vi "SLM Control.vi"() -> ()   [LabVIEW 2014]
uses:
  Controls/SLM General Settings.ctl
  Controls/Holo Settings.ctl
panel:
  in  "Exit":bool
  in  "Holo 2":T1={"Top Hat"=FALSE, "Modes"=[], "Vortex"=FALSE, "Clockwise"=FALSE, "X"=-200.0, "Y"=0.0, "Holo ON"=TRUE, "Scan"=FALSE} {"Modes"."Amplititute" step=0.05}
  out "Intensity Graph":u8[][](graph)
  in  "Holo 1":T1={"Top Hat"=FALSE, "Modes"=[], "Vortex"=FALSE, "Clockwise"=FALSE, "X"=200.0, "Y"=0.0, "Holo ON"=TRUE, "Scan"=FALSE} {"Modes"."Amplititute" step=0.05}
  in  "General settings":T2={"Holo size (pixels)"=300, "Top hat radius"=0.5, "Number of modes"=20, "Bkg gradient X"=40.0, "Bkg gradient Y"=40.0, "Flat"=FALSE, "Mode Matrix"=1} {"Mode Matrix" items=["Unit Matrix", "Unit Matrix_AbbNames"]; "Top hat radius" min=0.0 max=0.99 step=0.05 format="%.3f"}
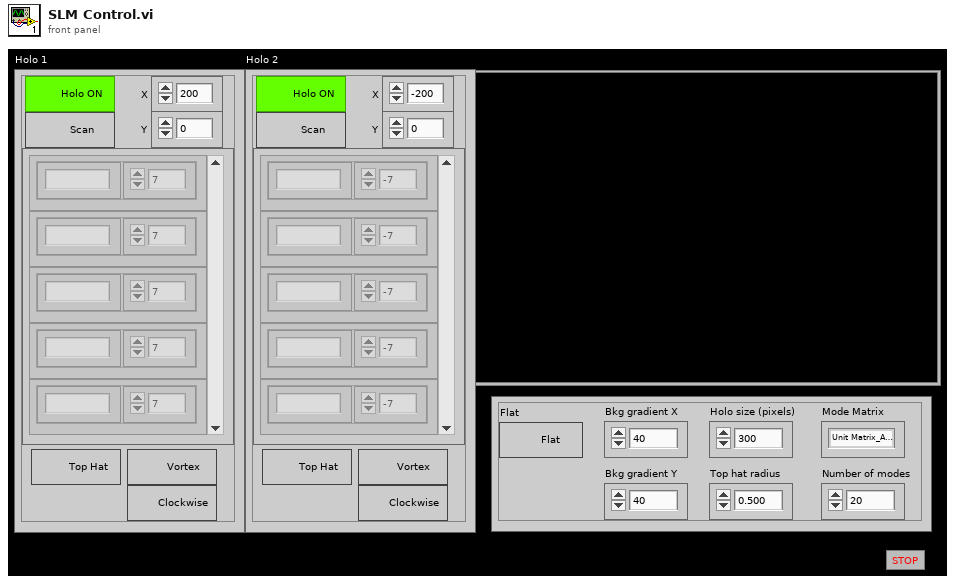
[diagram p1: front panel]
types:
  T1 = typedef "Holo Settings.ctl" = cluster{"Top Hat":bool, "Modes":cluster{"Mode ID":string, "Amplititute":dbl}[], "Vortex":bool, "Clockwise":bool, "X":dbl, "Y":dbl, "Holo ON":bool, "Scan":bool}
  T2 = typedef "SLM General Settings.ctl" = cluster{"Holo size (pixels)":i32, "Top hat radius":dbl, "Number of modes":i32, "Bkg gradient X":dbl, "Bkg gradient Y":dbl, "Flat":bool, "Mode Matrix":u16}
  T3 = cluster{"Holo size (pixels)":bool, "Top hat radius":bool, "Number of modes":bool, "Bkg gradient X":bool, "Bkg gradient Y":bool, "Flat":bool, "Mode Matrix":bool}
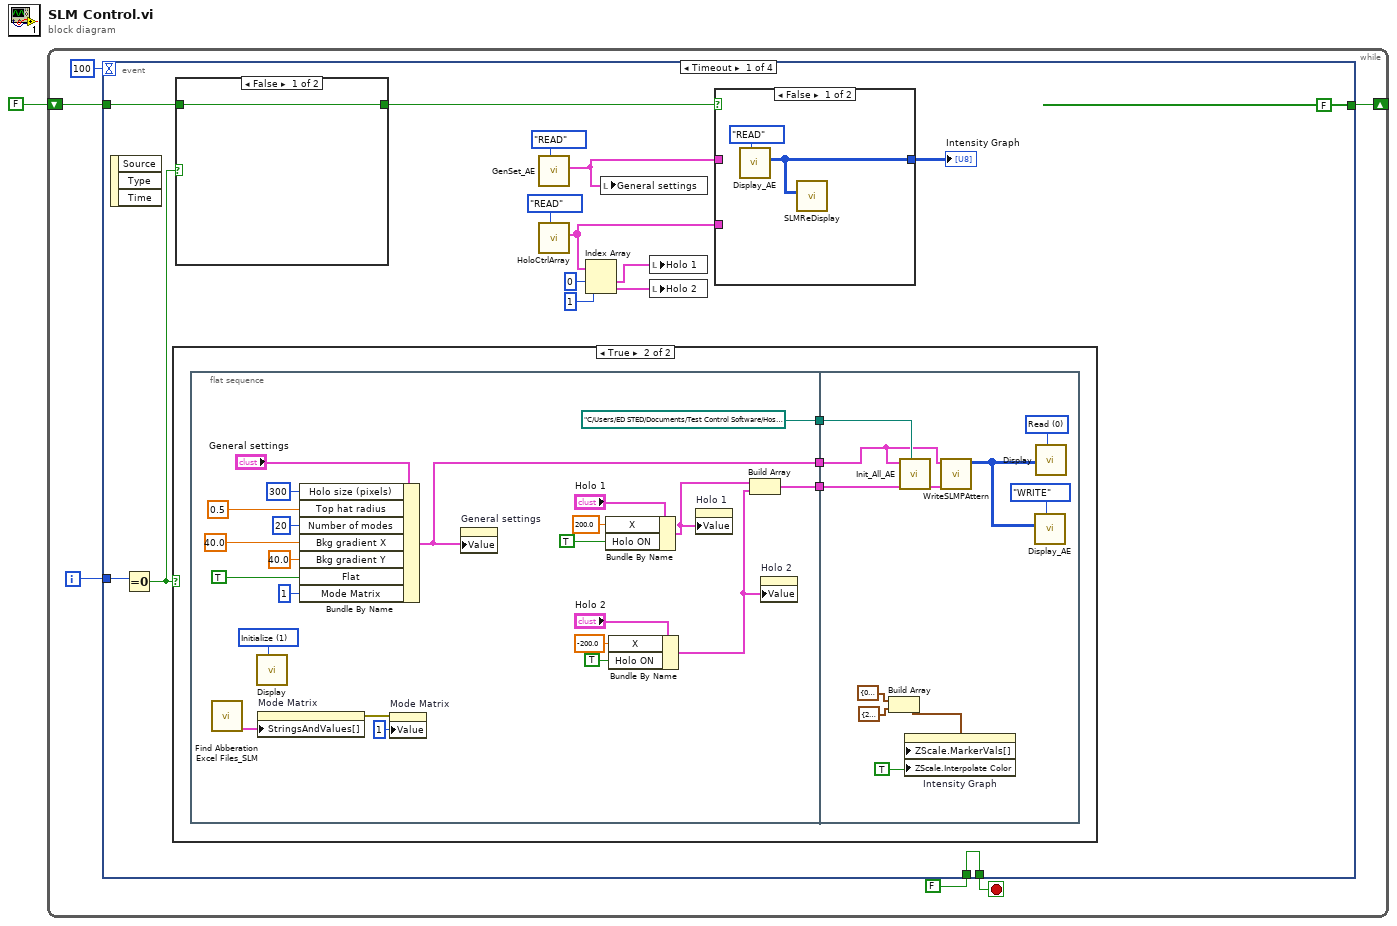
[diagram p0: block diagram]
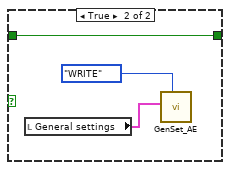
[diagram p2: hidden frame]
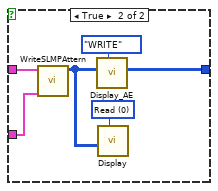
[diagram p3: hidden frame]
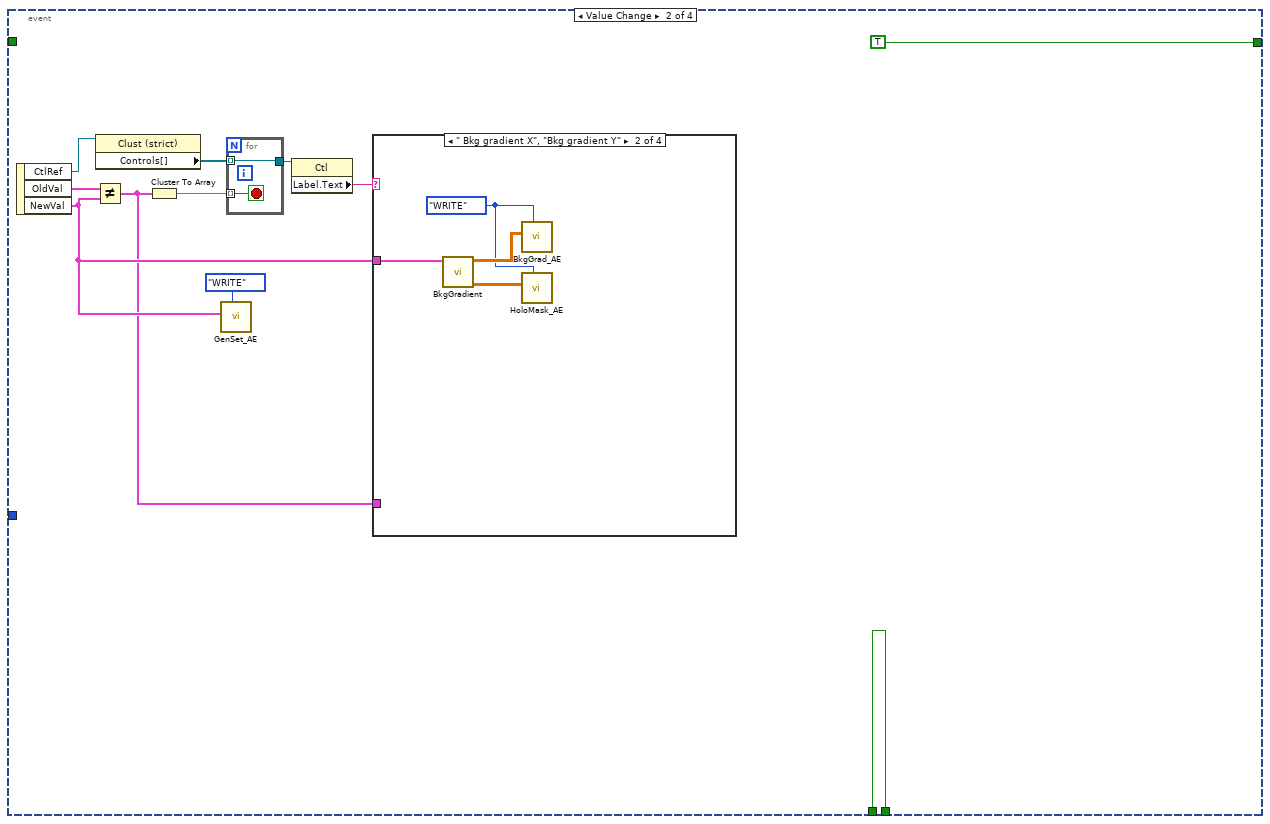
[diagram p5: hidden frame]
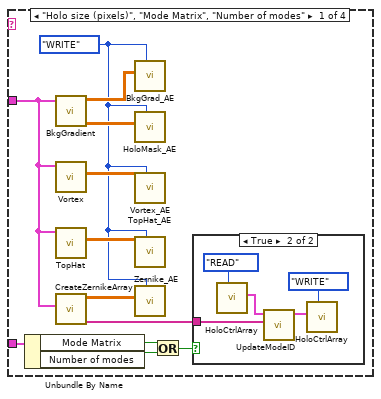
[diagram p6: hidden frame]
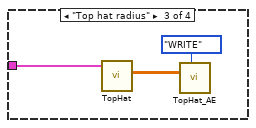
[diagram p8: hidden frame]
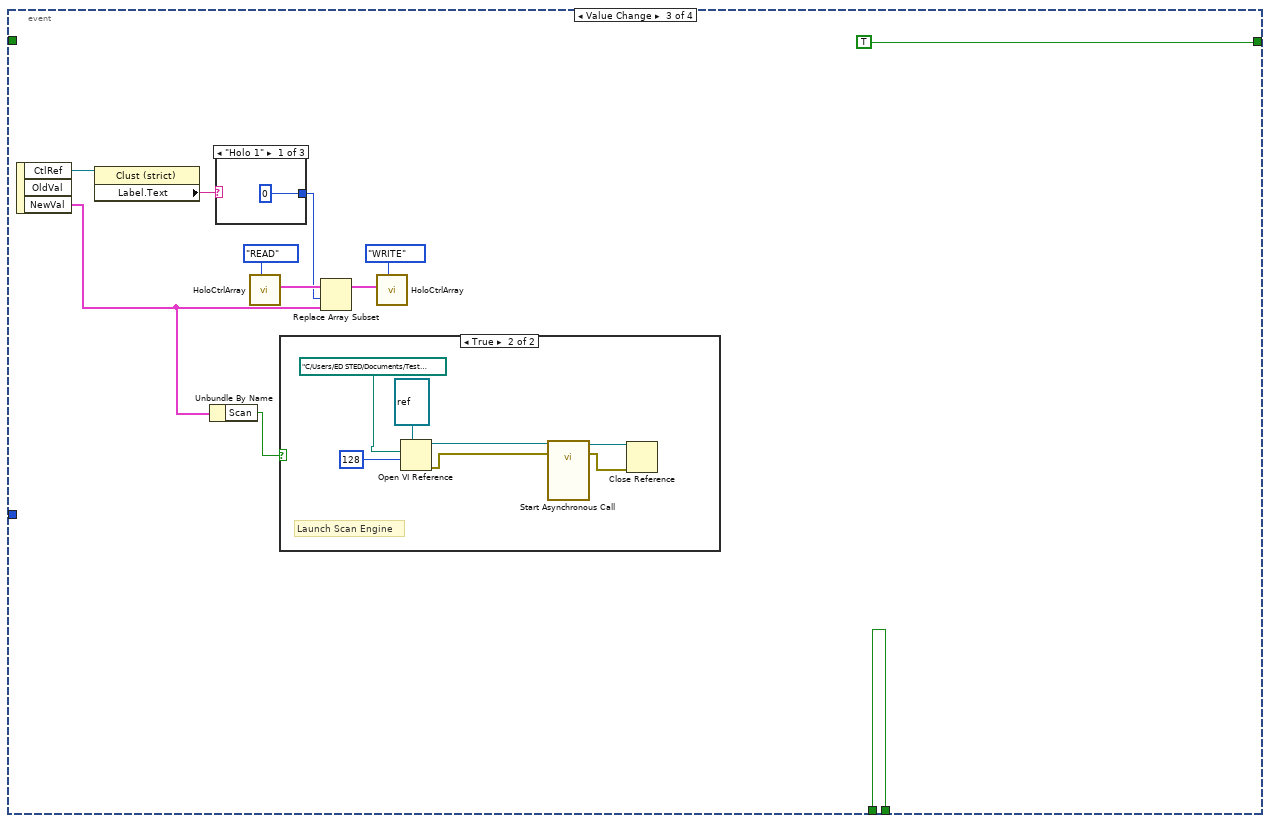
[diagram p10: hidden frame]
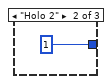
[diagram p12: hidden frame]
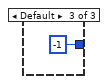
[diagram p13: hidden frame]
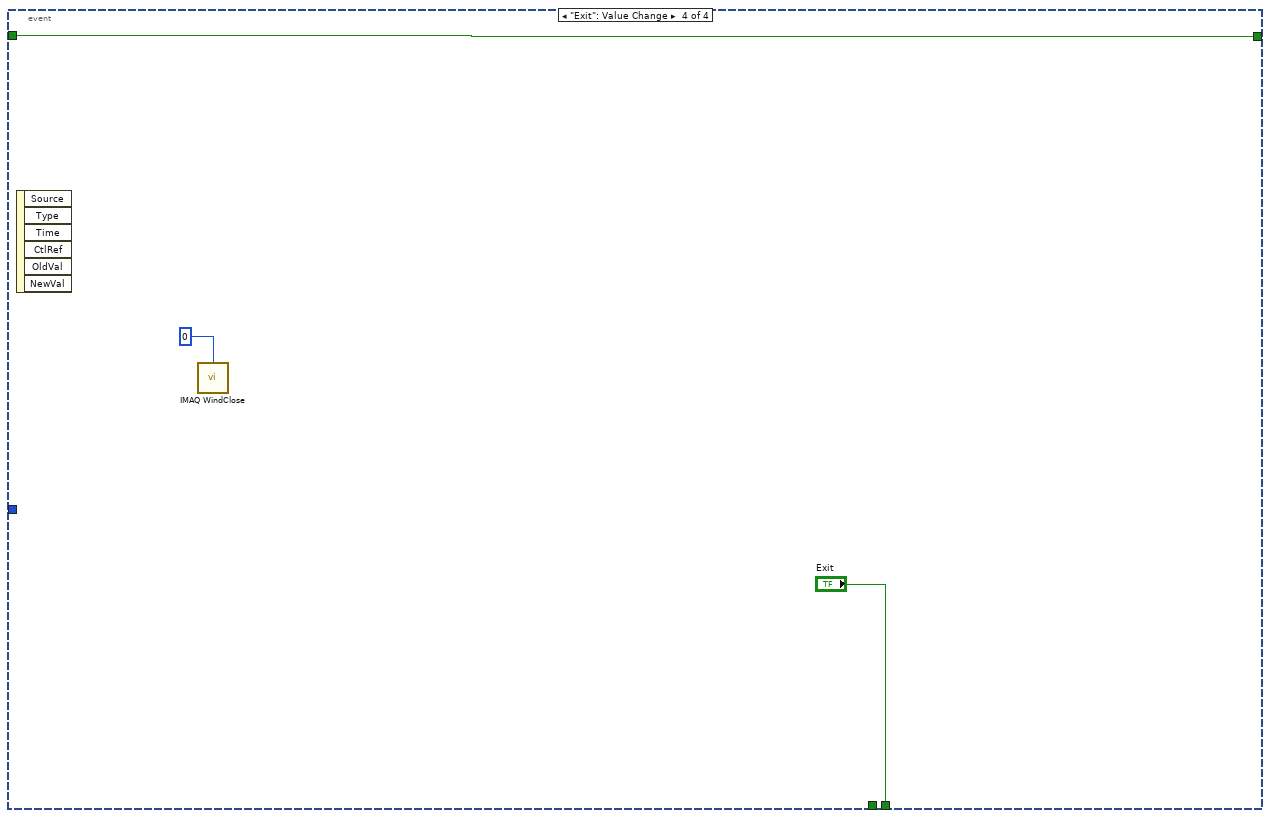
[diagram p14: hidden frame]
diagram:
  n1 = while {
    shift-right: [w4] -> _
    shift-left: FALSE -> [w5]
    i -> [w6]
    stop <- w3 stop-if-true
    n2 = event shown="[0] Timeout" {
      selector: _ -> [_ _ _ _]
      dyn-events: _ -> [_ _ _ _]
      timeout: 100 -> [_ _ _ _]
      tunnel: w6 -> [w22 _ _ _]
      tunnel: w5 -> [w10 _ _ w131]
      tunnel: [FALSE TRUE TRUE w131] -> w4
      tunnel: [w11 w73 w111 "Exit"] -> w3
      tunnel: FALSE -> [w11 w73 w111 _]
      event Timeout {
        n3 = event-data() -> ()  [unwired: 1 in, 3 out]
        n4 = Equal To 0?(x=w22) -> (x = 0?=w8:bool)
        n5 = case shown="True" w8 {
          frame False {
          }
          frame True {
            n6 = flat-sequence {
              tunnel: [w40] -> w37
              tunnel: [w56] -> w36
              tunnel: [path "C:/Users/ED STED/Documents/Test Control Software/Host VIs/SLM/Flatness Correction LSH0700935/CAL_LSH0700935_770nm.bmp" ("Flat File Path")] -> w35
              tunnel: w37 -> [w63]
              tunnel: w36 -> [w71]
              tunnel: w35 -> [w68]
              frame #0 {
                w57 = u16 1 items=["Read", "Initialize"] ("Action")
                n7 = call "Find Abberation Excel Files_SLM.vi"() -> ("Ring Menu"=w60:cluster{"result string":string, i32}[])  [unwired: 10 in, 1 out]
                n8 = call "Display.vi"("Action"=w57) -> ()  [unwired: 10 in, 1 out]
                n9 = property on="Mode Matrix" class="Ring (strict)"("StringsAndValues[]"=w60) -> (error out=w59:errorcluster)  [unwired: 2 in, 1 out]
                n10 = Bundle By Name(cluster="General settings", "Holo size (pixels)"=300, "Top hat radius"=0.5, "Number of modes"=20, "Bkg gradient X"=40.0, "Bkg gradient Y"=40.0, "Flat"=TRUE, "Mode Matrix"=u16 1) -> (w40:T2)
                n11 = property on="Mode Matrix" class="Ring (strict)"(error in=w59, "Value"=u16 1) -> ()  [unwired: 1 in, 2 out]
                n12 = property on="General settings" class="Clust (strict)"("Value"=w40) -> ()  [unwired: 2 in, 2 out]
                n13 = Bundle By Name(cluster="Holo 1", "X"=200.0, "Holo ON"=TRUE) -> (w44:T1)
                n14 = Bundle By Name(cluster="Holo 2", "X"=-200.0, "Holo ON"=TRUE) -> (w41:T1)
                n15 = property on="Holo 1" class="Clust (strict)"("Value"=w44) -> ()  [unwired: 2 in, 2 out]
                n16 = Build Array(w44, w41) -> (w56:T1[])
                n17 = property on="Holo 2" class="Clust (strict)"("Value"=w41) -> ()  [unwired: 2 in, 2 out]
              }
              frame #1 {
                w70 = u16 0 items=["Read", "Initialize"] ("Action")
                n18 = Build Array(cluster{dbl, u32} {0.0, 0}, cluster{dbl, u32} {255.0, 16448250}) -> (w64:cluster{dbl, u32}[])
                n19 = call "Init_All_AE.vi"("Flat File Path"=w68, "HoloArray In"=w71, "General settings"=w63) -> ("Holo Array Out"=w69:T1[])  [unwired: 8 in]
                n20 = property on="Intensity Graph" class="IntGraph (strict)"("ZScale.MarkerVals[]"=w64, "ZScale.Interpolate Color"=TRUE ("Z Scale.Interpolate Color")) -> ()  [unwired: 2 in, 2 out]
                n21 = call "WriteSLMPAttern.vi"("Holo Array"=w69, "General settings"=w63) -> ("Display Array"=w61:u8[][])  [unwired: 9 in]
                n22 = call "Display_AE.vi"("Action"=enum16{"READ", "WRITE"}."WRITE", "Display Array In"=w61) -> ()  [unwired: 9 in, 1 out]
                n23 = call "Display.vi"("Action"=w70, "displayed matrix"=w61) -> ()  [unwired: 9 in, 1 out]
              }
            }
          }
        }
        n24 = case shown="False" w8 {
          tunnel: w10 -> [w23 w26]
          tunnel: [w23 w26] -> w9
          frame False {
          }
          frame True {
            n25 = local read "General settings"() -> (w24:T2)
            n26 = call "GenSet_AE.vi"("Enum"=enum16{"READ", "WRITE"}."WRITE", "General settings"=w24) -> ()  [unwired: 9 in, 1 out]
          }
        }
        n27 = call "GenSet_AE.vi"("Enum"=enum16{"READ", "WRITE"}."READ") -> ("General settings Out"=w18:T2)  [unwired: 10 in]
        n28 = call "HoloCtrlArray.vi"("Action"=enum16{"READ", "WRITE"}."READ") -> ("Holo Array Out"=w17:T1[])  [unwired: 10 in]
        n29 = Index Array(array=w17, index #1=0 ("index"), index #2=1 ("index")) -> (element #1=w16:T1, element #2=w15:T1)
        n30 = local write "General settings"(w18) -> ()
        n31 = local write "Holo 1"(w16) -> ()
        n32 = local write "Holo 2"(w15) -> ()
        n33 = case shown="False" w9 {
          tunnel: w18 -> [_ w34]
          tunnel: w17 -> [_ w33]
          tunnel: [w27 w29] -> w12
          frame False {
            n34 = call "Display_AE.vi"("Action"=enum16{"READ", "WRITE"}."READ") -> ("Display Array Out"=w27:u8[][])  [unwired: 10 in]
            n35 = call "SLMReDisplay.vi"("displayed matrix"=w27) -> ()  [unwired: 11 in]
          }
          frame True {
            w32 = u16 0 items=["Read", "Initialize"] ("Action")
            n36 = call "WriteSLMPAttern.vi"("Holo Array"=w33, "General settings"=w34) -> ("Display Array"=w31:u8[][])  [unwired: 9 in]
            n37 = call "Display_AE.vi"("Action"=enum16{"READ", "WRITE"}."WRITE", "Display Array In"=w31) -> ("Display Array Out"=w29:u8[][])  [unwired: 9 in]
            n38 = call "Display.vi"("Action"=w32, "displayed matrix"=w31) -> ()  [unwired: 9 in, 1 out]
          }
        }
        "Intensity Graph" <- w12
      }
      event Value Change {
        n39 = event-data() -> ("CtlRef"=w81:refnum<vi>, "OldVal"=w82:T2, "NewVal"=w74:T2)  [unwired: 1 in]
        n40 = Not Equal?(x=w82, y=w74) -> (x != y?=w72:T3)
        n41 = property class="Clust (strict)"(reference=w81) -> ("Controls[]"=w80:refnum<vi>[])  [unwired: 1 in, 2 out]
        n42 = Cluster To Array(cluster=w72) -> (array=w79:bool[])
        n43 = call "GenSet_AE.vi"("Enum"=enum16{"READ", "WRITE"}."WRITE", "General settings"=w74) -> ()  [unwired: 9 in, 1 out]
        n44 = for {
          tunnel: [w108] -> w78
          tunnel: w80 -> [w108] mode=indexing
          tunnel: w79 -> [w107] mode=indexing
          stop <- w107 stop-if-true
        }
        n45 = property class="Ctl"(reference=w78) -> ("Label.Text"=w77:string)  [unwired: 1 in, 2 out]
        n46 = case shown="\" Bkg gradient X\", \"Bkg gradient Y\"" w77 {
          tunnel: w74 -> [w88 w100 w106 _]
          tunnel: w72 -> [w86 _ _ _]
          frame "Holo size (pixels)", "Mode Matrix", "Number of modes" {
            w87 = enum16{"READ", "WRITE"}."WRITE" ("Action")
            n47 = Unbundle By Name(w86) -> ("Mode Matrix"=w85:bool, "Number of modes"=w84:bool)
            n48 = call "BkgGradient.vi"("General settings"=w88) -> ("Holo mask"=w93:dbl[][], "gradient"=w94:dbl[][])  [unwired: 9 in]
            n49 = call "Vortex.vi"("General settings"=w88) -> ("Vortex"=w91:dbl[][])  [unwired: 10 in]
            n50 = call "TopHat.vi"("General settings"=w88) -> ("TopHat"=w92:dbl[][])  [unwired: 10 in]
            n51 = call "CreateZernikeArray.vi"("General settings"=w88) -> ("Mode IDs"=w89:string[], "Modes Out"=w90:dbl[][][])  [unwired: 9 in]
            n52 = call "BkgGrad_AE.vi"("Action"=w87, "BkgGrad In"=w94) -> ()  [unwired: 9 in, 1 out]
            n53 = call "HoloMask_AE.vi"("Action"=w87, "HoloMask In"=w93) -> ()  [unwired: 9 in, 1 out]
            n54 = call "Vortex_AE.vi"("Action"=w87, "Vortex In"=w91) -> ()  [unwired: 9 in, 1 out]
            n55 = call "TopHat_AE.vi"("Action"=w87, "TopHat In"=w92) -> ()  [unwired: 9 in, 1 out]
            n56 = call "Zernike_AE.vi"("Action"=w87, "Zernike In"=w90) -> ()  [unwired: 9 in, 1 out]
            n57 = Or(x=w85, y=w84) -> (x .or. y?=w83:bool)
            n58 = case shown="True" w83 {
              tunnel: w89 -> [_ w99]
              frame False {
              }
              frame True {
                n59 = call "HoloCtrlArray.vi"("Action"=enum16{"READ", "WRITE"}."READ") -> ("Holo Array Out"=w98:T1[])  [unwired: 10 in]
                n60 = call "UpdateModeID.vi"("Mode IDs"=w99, "Array in"=w98) -> ("Array out"=w95:T1[])  [unwired: 9 in]
                n61 = call "HoloCtrlArray.vi"("Action"=enum16{"READ", "WRITE"}."WRITE", "Holo Array In"=w95) -> ()  [unwired: 9 in, 1 out]
              }
            }
          }
          frame " Bkg gradient X", "Bkg gradient Y" {
            w101 = enum16{"READ", "WRITE"}."WRITE" ("Action")
            n62 = call "BkgGradient.vi"("General settings"=w100) -> ("Holo mask"=w102:dbl[][], "gradient"=w103:dbl[][])  [unwired: 9 in]
            n63 = call "BkgGrad_AE.vi"("Action"=w101, "BkgGrad In"=w103) -> ()  [unwired: 9 in, 1 out]
            n64 = call "HoloMask_AE.vi"("Action"=w101, "HoloMask In"=w102) -> ()  [unwired: 9 in, 1 out]
          }
          frame "Top hat radius" {
            n65 = call "TopHat.vi"("General settings"=w106) -> ("TopHat"=w105:dbl[][])  [unwired: 10 in]
            n66 = call "TopHat_AE.vi"("Action"=enum16{"READ", "WRITE"}."WRITE", "TopHat In"=w105) -> ()  [unwired: 9 in, 1 out]
          }
          frame Default {
          }
        }
      }
      event Value Change {
        n67 = event-data() -> ("CtlRef"=w116:refnum<vi>, "NewVal"=w110:T1)  [unwired: 1 in, 1 out]
        n68 = property class="Clust (strict)"(reference=w116) -> ("Label.Text"=w115:string)  [unwired: 1 in, 2 out]
        n69 = Unbundle By Name(w110) -> ("Scan"=w109:bool)
        n70 = case shown="\"Holo 1\"" w115 {
          tunnel: [0 1 -1] -> w114
          frame "Holo 1" {
          }
          frame "Holo 2" {
          }
          frame Default {
          }
        }
        n71 = call "HoloCtrlArray.vi"("Action"=enum16{"READ", "WRITE"}."READ") -> ("Holo Array Out"=w117:T1[])  [unwired: 10 in]
        n72 = case shown="True" w109 {
          frame False {
          }
          frame True {
            # "Launch Scan Engine"
            n73 = Open VI Reference(type specifier VI Refnum (for type only)=refnum<vi> refnum, vi path=path "C:/Users/ED STED/Documents/Test Control Software/Host VIs/SLM/Scan/ScanMode_SLM.vi", options=128) -> (vi reference=w121:refnum<vi>, error out=w120:errorcluster)  [unwired: 3 in]
            n74 = call-by-ref "Start Asynchronous Call"(reference=w121, error in=w120) -> (reference out=w123:refnum<vi>, error out=w122:errorcluster)  [unwired: 12 in]
            n75 = Close Reference(reference=w123, error in (no error)=w122) -> ()  [unwired: 1 out]
          }
        }
        n76 = Replace Array Subset(array=w117, new element=w110, index=w114) -> (w112:T1[])
        n77 = call "HoloCtrlArray.vi"("Action"=enum16{"READ", "WRITE"}."WRITE", "Holo Array In"=w112) -> ()  [unwired: 9 in, 1 out]
      }
      event "Exit": Value Change {
        n78 = event-data() -> ()  [unwired: 1 in, 6 out]
        n79 = call "IMAQ WindClose"("Window Number (0...15)"=0) -> ()  [unwired: 2 in, 4 out]
      }
    }
  }
